vi "array dim size (3d).vi"(1 "dim":i32, 2 "array":dbl[][][](array[numeric])) -> (0 "dim size":i32)   [LabVIEW 2012, in "common.lvlib"]
uses:
  common.lvlib
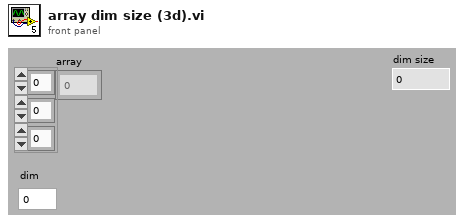
[diagram p1: front panel]
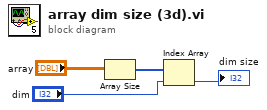
[diagram p0: block diagram]
diagram:
  n1 = Array Size(array="array") -> (size(s)=w3:i32[])
  n2 = Index Array(array=w3, index="dim") -> (element=→"dim size":i32)
